vi "GTH-V2.CurrentMeter.vi"(8 "Error In":errorcluster caption="错误输入", 10 "Calibration_Para":dbl[][](array[numeric]), 11 "VISA资源输入":refnum<visa-resource-name>) -> (0 "Error Out":errorcluster caption="错误输出", 1 "波形图":waveform(dbl)(graph), 2 "DataOut":cluster{"均方根电流(mA)":dbl, "均值电流(mA)":dbl}, 3 "OK?":bool)   [LabVIEW 2012, in "Lib_UEL.ATE.lvlib" / "STM32-CoreBD.lvlib"]
uses:
  STM32-CoreBD.lvlib
panel:
  out "布尔":bool
  # "Version History\nV1.0.0,2015-8-11, 初始版本, 硬件GTH-V2"
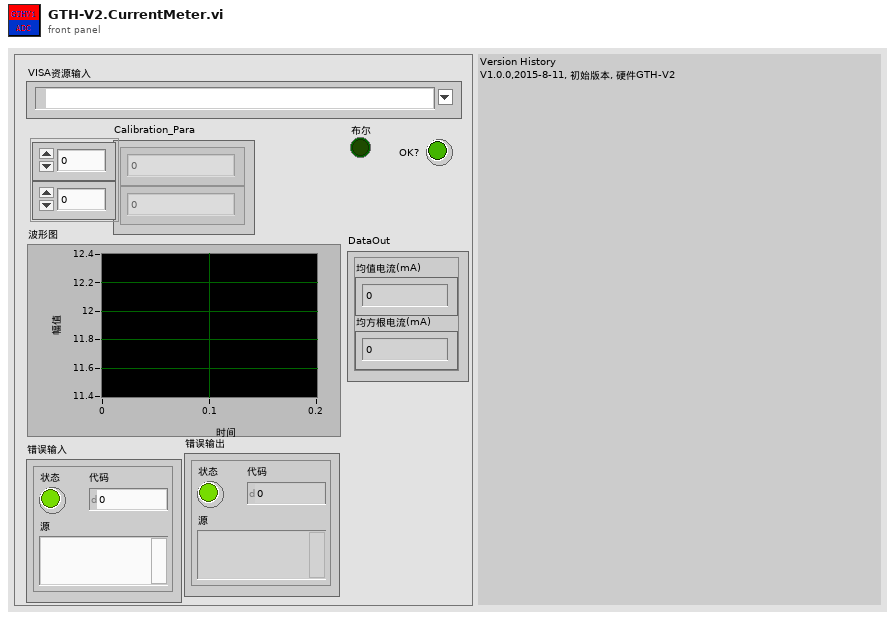
[diagram p1: front panel]
types:
  T1 = enum16{"Read_Version", "Read_PID", "Read_CalibrationInfo", "Read_C_Value_ADC_ChanA", "Read_C_Value_ADC_ChanB", "Read_C_Value_Current", "Read_C_Value_DAC", "Write_CalibrationInfo", "Write_C_Value_ADC_ChanA", "Write_C_Value_ADC_ChanB", "Write_C_Value_Current", "Write_C_Value_DAC"}
  T2 = enum16{"RelayA1", "RelayA2", "RelayA3", "RelayA4", "RelayA5", "RelayA6", "RelayA7", "RelayA8", "RelayA9", "RelayA10", "RelayB1", "RelayB2", "RelayB3", "RelayB4", "RelayB5", "RelayB6", "RelayB7", "RelayB8", "RelayB9", "RelayB10", "ADC1", "ADC2", "ADC3", "DAC1"}
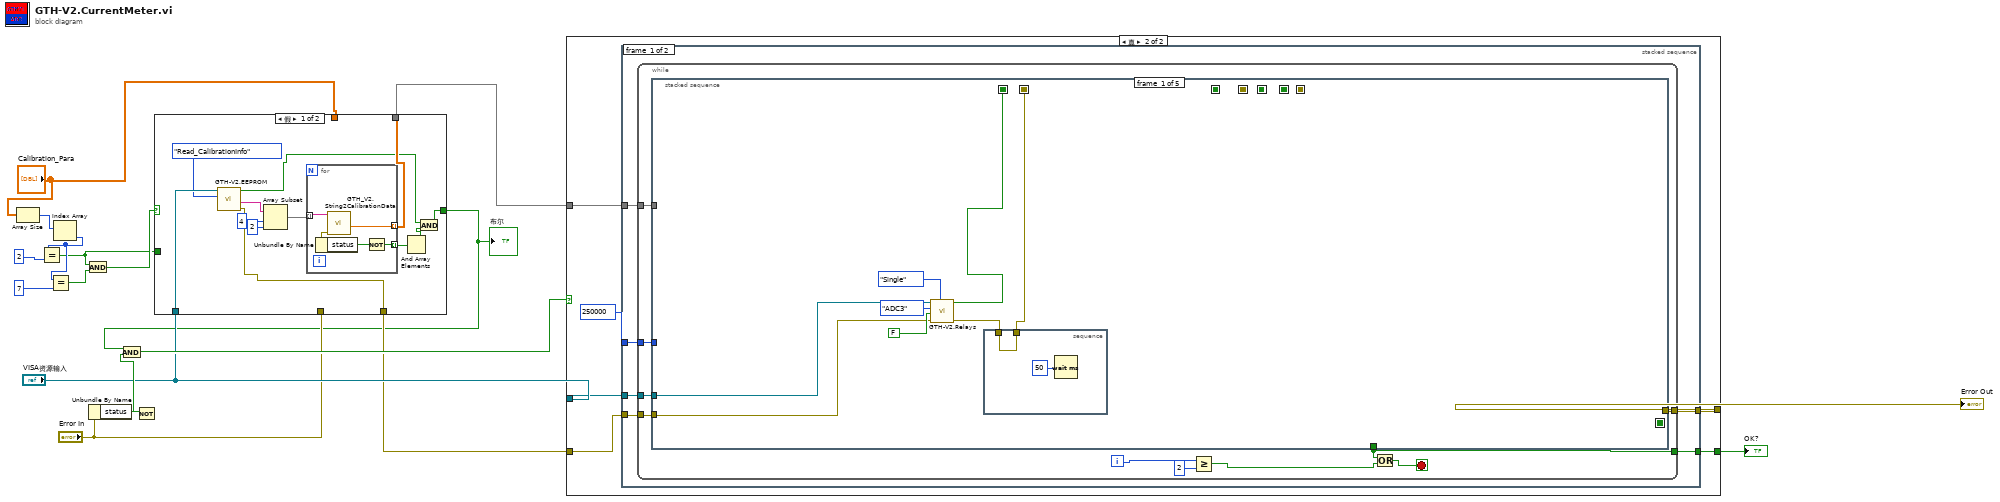
[diagram p0: block diagram]
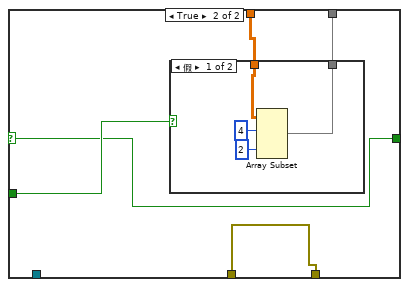
[diagram p2: hidden frame]
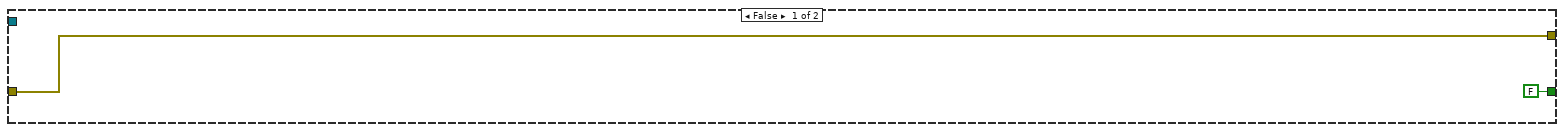
[diagram p4: hidden frame]
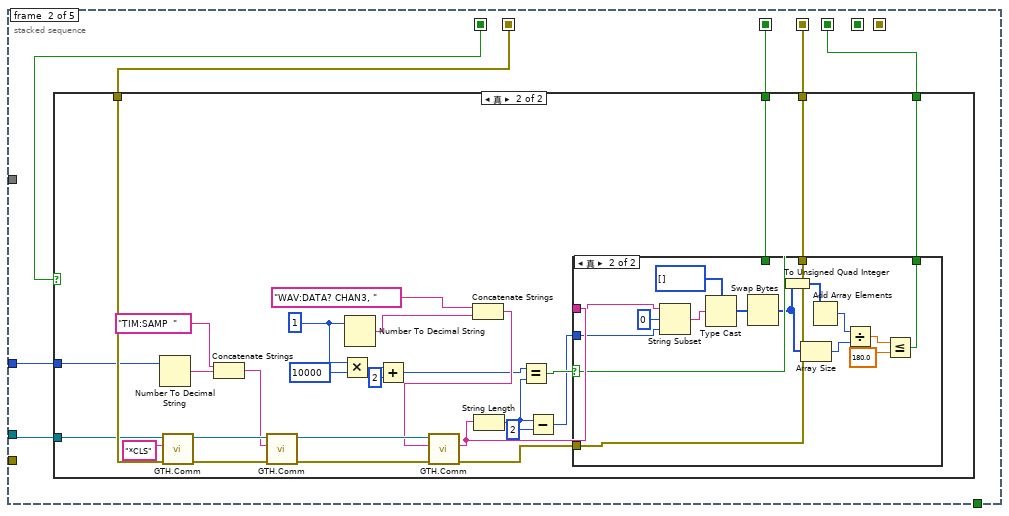
[diagram p5: hidden frame]
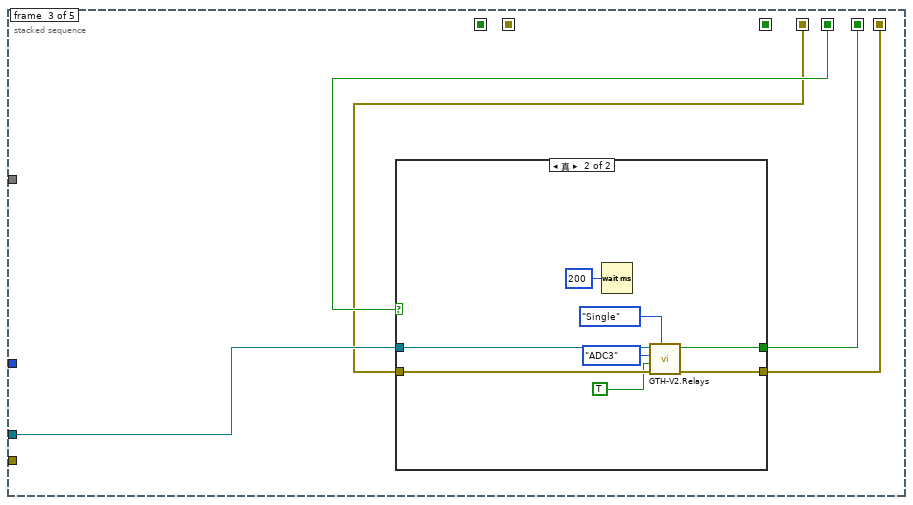
[diagram p8: hidden frame]
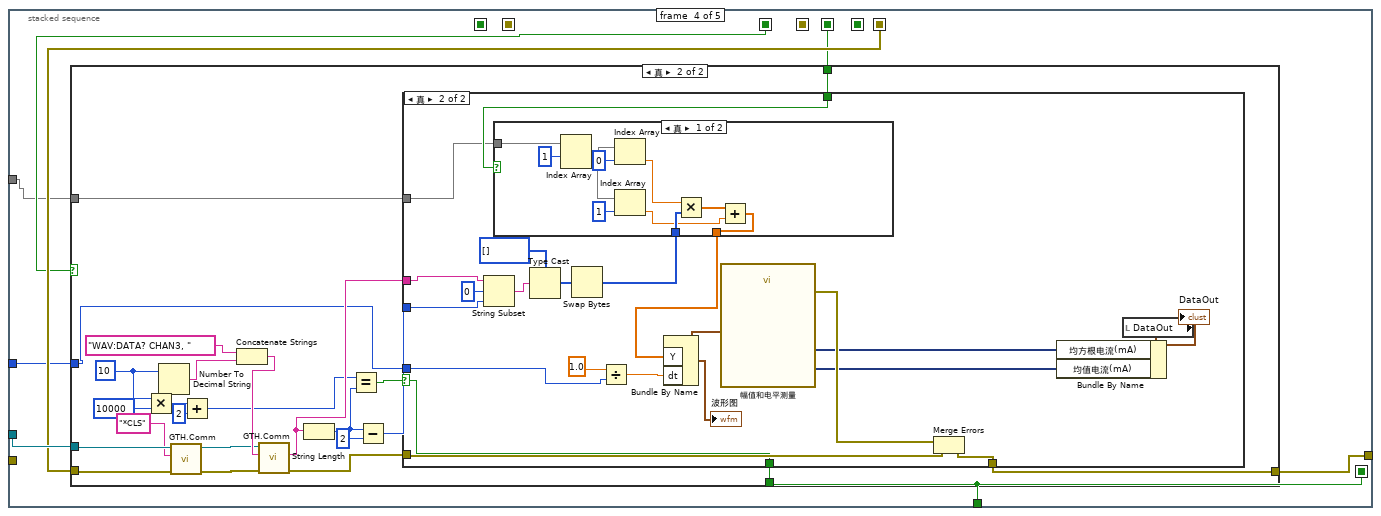
[diagram p10: hidden frame]
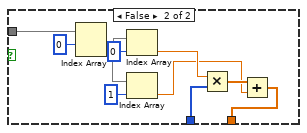
[diagram p13: hidden frame]
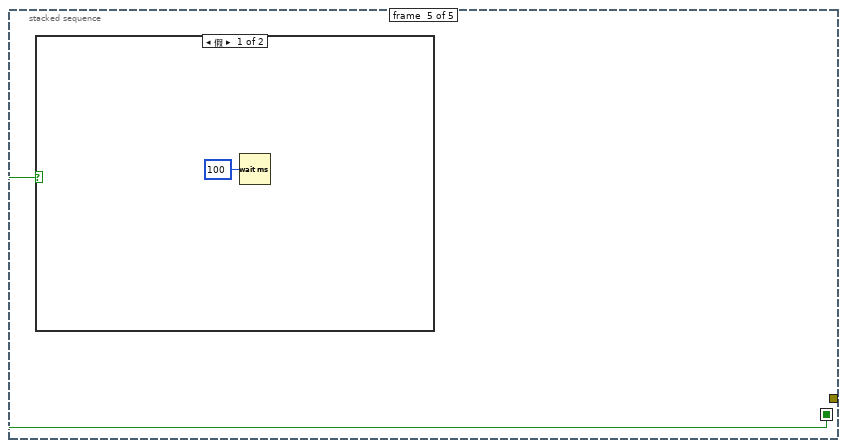
[diagram p14: hidden frame]
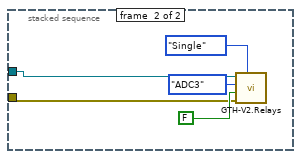
[diagram p16: hidden frame]
diagram:
  n1 = Array Size(array="Calibration_Para") -> (size(s)=w12:i32[])
  n2 = Index Array(array=w12) -> (element=w5:i32)  [unwired: 1 in]
  n3 = Equal?(x=w5, y=2) -> (x = y?=w1:bool)
  n4 = Equal?(x=w5, y=7) -> (x = y?=w3:bool)
  n5 = And(x=w1, y=w3) -> (x .and. y?=w2:bool)
  n6 = Unbundle By Name("Error In") -> ("status"=w16:bool)
  n7 = Not(x=w16) -> (.not. x?=w13:bool)
  n8 = case shown="假" w2 {
    selector: w2 -> [_ w36]
    tunnel: [w25 w39] -> w9
    tunnel: "Calibration_Para" -> [_ w38]
    tunnel: "VISA资源输入" -> [w30 _]
    tunnel: [w19 w36] -> w6
    tunnel: [w24 w40] -> w7
    tunnel: "Error In" -> [_ w40]
    tunnel: w1 -> [_ w37]
    frame False {
      n9 = call "GTH-V2.EEPROM.vi"("CMD"=T1."Read_CalibrationInfo", "VISA资源输入"=w30) -> ("Error Out"=w24:errorcluster, "Calibration_Value_Out"=w28:string[], "OK?"=w20:bool)  [unwired: 6 in, 1 out]
      n10 = Array Subset(array=w28, index=4 ("索引"), length=2 ("长度")) -> (w26:string[])
      n11 = for {
        tunnel: w26 -> [w35] mode=indexing
        tunnel: [w34] -> w25 mode=indexing
        tunnel: [w31] -> w22 mode=indexing
        n12 = call "GTH_V2.String2CalibrationData.vi"("String"=w35) -> ("错误输出"=w33:errorcluster, "Para"=w34:dbl[])  [unwired: 5 in, 4 out]
        n13 = Unbundle By Name(w33) -> ("status"=w32:bool)
        n14 = Not(x=w32) -> (.not. x?=w31:bool)
      }
      n15 = And Array Elements(Boolean array=w22) -> (logical AND=w21:bool)
      n16 = And(x=w20, y=w21) -> (x .and. y?=w19:bool)
    }
    frame True {
      n17 = case shown="假" w37 {
        tunnel: [w41 w45] -> w39
        tunnel: w38 -> [w44 w45]
        frame False {
          n18 = Array Subset(array=w44, index (row)=4 ("索引"), length (row)=2 ("长度")) -> (w41:dbl[][])  [unwired: 2 in]
        }
        frame True {
        }
      }
    }
  }
  "布尔" <- w6
  n19 = And(x=w6, y=w13) -> (x .and. y?=w14:bool)
  n20 = case shown="真" w14 {
    tunnel: [w46 w53] -> w18
    tunnel: "VISA资源输入" -> [_ w52]
    tunnel: [FALSE w51] -> w17
    tunnel: w7 -> [w46 w50]
    tunnel: w9 -> [_ w49]
    frame False {
    }
    frame True {
      n21 = stacked-sequence {
        tunnel: [w59 _] -> w53
        tunnel: w52 -> [w58 w230]
        tunnel: w50 -> [w57 w229]
        tunnel: [w56 _] -> w51
        tunnel: w49 -> [w55 _]
        tunnel: u32 250000 ("y") -> [w54 _]
        frame #0 {
          n22 = while {
            tunnel: [w66] -> w59
            tunnel: w58 -> [w69]
            tunnel: w57 -> [w68]
            tunnel: [w62] -> w56
            tunnel: w55 -> [w61]
            tunnel: w54 -> [w60]
            i -> [w65]
            stop <- w67 stop-if-true
            n23 = stacked-sequence {
              seq-local: [_ _ _ w154 _] -> [_ _ _ _ w227]
              seq-local: [_ w86 _ _ _] -> [_ _ w136 _ _]
              seq-local: [_ w85 _ _ _] -> [_ _ _ w151 _]
              seq-local: [_ w84 _ _ _] -> [_ _ w138 w152 _]
              seq-local: [w72 _ _ _ _] -> [_ w81 _ _ _]
              seq-local: [w71 _ _ _ _] -> [_ w83 _ _ _]
              seq-local: [_ _ w135 _ _] -> [_ _ _ _ _]
              seq-local: [_ _ w134 _ _] -> [_ _ _ w153 _]
              tunnel: w69 -> [w77 w82 w137 w156 _]
              tunnel: w68 -> [w73 _ _ _ _]
              tunnel: [_ _ _ w155 _] -> w66
              tunnel: [_ _ _ w154 _] -> w62
              tunnel: w61 -> [_ _ _ w150 _]
              tunnel: w60 -> [_ w80 _ w149 _]
              frame #0 {
                n24 = call "GTH-V2.Relays.vi"("CMD"=enum16{"All", "ChanA", "ChanB", "Single"}."Single", "Error In"=w73, "ON/FF"=FALSE, "Para"=T2."ADC3", "VISA资源输入"=w77) -> ("Error Out"=w70:errorcluster, "OK?"=w72:bool)  [unwired: 4 in, 1 out]
                n25 = stacked-sequence {
                  tunnel: [w78] -> w71
                  tunnel: w70 -> [w78]
                  frame #0 {
                    n26 = Wait (ms)(milliseconds to wait=u32 50 ("等待时间（毫秒）")) -> ()  [unwired: 1 out]
                  }
                }
              }
              frame #1 {
                n27 = case shown="真" w81 {
                  selector: w81 -> [w88 _]
                  tunnel: [w87 w97] -> w86
                  tunnel: [w88 w96] -> w85
                  tunnel: [w88 w95] -> w84
                  tunnel: w83 -> [w87 w94]
                  tunnel: w82 -> [_ w93]
                  tunnel: w80 -> [_ w92]
                  frame False {
                  }
                  frame True {
                    w99 = u32 1 ("y")
                    n28 = Number To Decimal String(number=w92) -> (decimal integer string=w91:string)  [unwired: 1 in]
                    n29 = call "GTH.Comm.vi"("Error In"=w94, "SCPI CMD"="*CLS" ("字符串"), "USB Port In"=w93) -> ("Error Out"=w114:errorcluster, "USB Port Out"=w115:refnum<visa-resource-name>)  [unwired: 3 in, 4 out]
                    n30 = Concatenate Strings("TIM:SAMP  " ("字符串"), w91) -> (w89:string)
                    n31 = call "GTH.Comm.vi"("Error In"=w114, "SCPI CMD"=w89, "USB Port In"=w115) -> ("Error Out"=w111:errorcluster, "USB Port Out"=w112:refnum<visa-resource-name>)  [unwired: 3 in, 4 out]
                    n32 = Multiply(x=w99, y=u32 10000) -> (x*y=w107:u32)
                    n33 = Number To Decimal String(number=w99) -> (decimal integer string=w113:string)  [unwired: 1 in]
                    n34 = Add(x=w107, y=u32 2) -> (x+y=w104:u32)
                    n35 = Concatenate Strings("WAV:DATA? CHAN3, " ("字符串"), w113) -> (w110:string)
                    n36 = call "GTH.Comm.vi"("Error In"=w111, "SCPI CMD"=w110, "USB Port In"=w112) -> ("Error Out"=w109:errorcluster, "Return"=w105:string)  [unwired: 3 in, 4 out]
                    n37 = String Length(string=w105) -> (length=w102:i32)
                    n38 = Equal?(x=w104, y=w102) -> (x = y?=w103:bool)
                    n39 = Subtract(x=w102, y=2) -> (x-y=w100:i32)
                    n40 = case shown="真" w103 {
                      selector: w103 -> [w117 w127]
                      tunnel: w109 -> [w118 w121]
                      tunnel: w105 -> [_ w130]
                      tunnel: w100 -> [_ w128]
                      tunnel: [w118 w121] -> w97
                      tunnel: [w117 w127] -> w96
                      tunnel: [w117 w122] -> w95
                      frame False {
                      }
                      frame True {
                        n41 = String Subset(string=w130, offset (0)=0 ("偏移量(0)"), length (rest)=w128) -> (substring=w131:string)
                        n42 = Type Cast(type=u16[] [], x=w131) -> (*(type *) &x=w132:u16[])
                        n43 = Swap Bytes(anything=w132) -> (byte swapped=w120:u16[])
                        n44 = To Unsigned Quad Integer(1:w120) -> (0:w119:u64[])
                        n45 = Array Size(array=w120) -> (size(s)=w125:i32)
                        n46 = Add Array Elements(numeric array=w119) -> (sum=w126:u64)
                        n47 = Divide(x=w126, y=w125) -> (x/y=w124:dbl)
                        n48 = Less Or Equal?(x=w124, y=180.0) -> (x <= y?=w122:bool)
                      }
                    }
                  }
                }
              }
              frame #2 {
                n49 = case shown="真" w138 {
                  selector: w138 -> [w140 _]
                  tunnel: w137 -> [_ w148]
                  tunnel: w136 -> [w139 w147]
                  tunnel: [w140 w143] -> w135
                  tunnel: [w139 w142] -> w134
                  frame False {
                  }
                  frame True {
                    n50 = Wait (ms)(milliseconds to wait=u32 200 ("等待时间（毫秒）")) -> ()  [unwired: 1 out]
                    n51 = call "GTH-V2.Relays.vi"("CMD"=enum16{"All", "ChanA", "ChanB", "Single"}."Single", "Error In"=w147, "ON/FF"=TRUE, "Para"=T2."ADC3", "VISA资源输入"=w148) -> ("Error Out"=w142:errorcluster, "OK?"=w143:bool)  [unwired: 4 in, 1 out]
                  }
                }
              }
              frame #3 {
                n52 = case shown="真" w151 {
                  selector: w151 -> [w158 _]
                  tunnel: w156 -> [_ w182]
                  tunnel: w153 -> [w157 w181]
                  tunnel: [w157 w167] -> w155
                  tunnel: [w158 w166] -> w154
                  tunnel: w152 -> [_ w161]
                  tunnel: w150 -> [_ w160]
                  tunnel: w149 -> [_ w159]
                  frame False {
                  }
                  frame True {
                    w165 = u32 10 ("y")
                    n53 = Multiply(x=w165, y=u32 10000) -> (x*y=w175:u32)
                    n54 = Number To Decimal String(number=w165) -> (decimal integer string=w179:string)  [unwired: 1 in]
                    n55 = call "GTH.Comm.vi"("Error In"=w181, "SCPI CMD"="*CLS" ("字符串"), "USB Port In"=w182) -> ("Error Out"=w162:errorcluster, "USB Port Out"=w163:refnum<visa-resource-name>)  [unwired: 3 in, 4 out]
                    n56 = Add(x=w175, y=u32 2) -> (x+y=w172:u32)
                    n57 = Concatenate Strings("WAV:DATA? CHAN3, " ("字符串"), w179) -> (w178:string)
                    n58 = call "GTH.Comm.vi"("Error In"=w162, "SCPI CMD"=w178, "USB Port In"=w163) -> ("Error Out"=w177:errorcluster, "Return"=w173:string)  [unwired: 3 in, 4 out]
                    n59 = String Length(string=w173) -> (length=w170:i32)
                    n60 = Equal?(x=w172, y=w170) -> (x = y?=w171:bool)
                    n61 = Subtract(x=w170, y=2) -> (x-y=w168:i32)
                    n62 = case shown="真" w171 {
                      selector: w171 -> [w183 w196]
                      tunnel: [w184 w202] -> w167
                      tunnel: w177 -> [w184 w201]
                      tunnel: w173 -> [_ w199]
                      tunnel: w168 -> [_ w197]
                      tunnel: [w183 w196] -> w166
                      tunnel: w161 -> [_ w191]
                      tunnel: w160 -> [_ w190]
                      tunnel: w159 -> [_ w185]
                      frame False {
                      }
                      frame True {
                        n63 = String Subset(string=w199, offset (0)=0 ("偏移量(0)"), length (rest)=w197) -> (substring=w200:string)
                        n64 = Type Cast(type=u16[] [], x=w200) -> (*(type *) &x=w205:u16[])
                        n65 = Swap Bytes(anything=w205) -> (byte swapped=w189:u16[])
                        n66 = case shown="真" w191 {
                          tunnel: w190 -> [w216 w226]
                          tunnel: w189 -> [w214 w224]
                          tunnel: [w212 w222] -> w188
                          frame True {
                            n67 = Index Array(array=w216, index (row)=1 ("索引")) -> (element=w211:dbl[])  [unwired: 1 in]
                            n68 = Index Array(array=w211, index=0 ("索引")) -> (element=w208:dbl)
                            n69 = Index Array(array=w211, index=1 ("索引")) -> (element=w207:dbl)
                            n70 = Multiply(x=w208, y=w214) -> (x*y=w213:dbl[])
                            n71 = Add(x=w213, y=w207) -> (x+y=w212:dbl[])
                          }
                          frame False {
                            n72 = Index Array(array=w226, index (row)=0 ("索引")) -> (element=w221:dbl[])  [unwired: 1 in]
                            n73 = Index Array(array=w221, index=0 ("索引")) -> (element=w218:dbl)
                            n74 = Index Array(array=w221, index=1 ("索引")) -> (element=w217:dbl)
                            n75 = Multiply(x=w218, y=w224) -> (x*y=w223:dbl[])
                            n76 = Add(x=w223, y=w217) -> (x+y=w222:dbl[])
                          }
                        }
                        n77 = Divide(x=1.0 ("y"), y=w185) -> (x/y=w192:dbl)
                        n78 = Bundle By Name("Y"=w188, "dt"=w192) -> (w194:waveform(dbl))  [unwired: 1 in]
                        "波形图" <- w194
                        n79 = call "幅值和电平测量"("Signals"=w194) -> ("Mean (DC)"=w187:dynamicdata, "RMS"=w186:dynamicdata, "error out"=w195:errorcluster)  [unwired: 12 in]
                        n80 = Merge Errors(w195, w201) -> (w202:errorcluster)
                        n81 = local read "DataOut"() -> (w203:cluster{"均方根电流(mA)":dbl, "均值电流(mA)":dbl})
                        n82 = Bundle By Name(cluster=w203, "均方根电流(mA)"=w186, "均值电流(mA)"=w187) -> (→"DataOut":cluster{"均方根电流(mA)":dbl, "均值电流(mA)":dbl})
                      }
                    }
                  }
                }
              }
              frame #4 {
                n83 = case shown="假" w227 {
                  frame False {
                    n84 = Wait (ms)(milliseconds to wait=u32 100 ("等待时间（毫秒）")) -> ()  [unwired: 1 out]
                  }
                  frame True {
                  }
                }
              }
            }
            n85 = Greater Or Equal?(x=w65, y=2) -> (x >= y?=w63:bool)
            n86 = Or(x=w62, y=w63) -> (x .or. y?=w67:bool)
          }
        }
        frame #1 {
          n87 = call "GTH-V2.Relays.vi"("CMD"=enum16{"All", "ChanA", "ChanB", "Single"}."Single", "Error In"=w229, "ON/FF"=FALSE, "Para"=T2."ADC3", "VISA资源输入"=w230) -> ()  [unwired: 4 in, 3 out]
        }
      }
    }
  }
  "Error Out" <- w18
  "OK?" <- w17
